vi "send.vi"(8 "error in (no error)":errorcluster, 10 "message":string, 11 "TCPConnection In":refnum<class "TCPConnection.lvclass">) -> (0 "error out":errorcluster, 3 "TCPConnection Out":refnum<class "TCPConnection.lvclass">)   [LabVIEW 2023, in "AbstractFactory.lvlib" / "TCPConnection.lvclass"]
uses:
  TCPConnection.lvclass
  TCPConnection.lvclass/TCPConnection.ctl
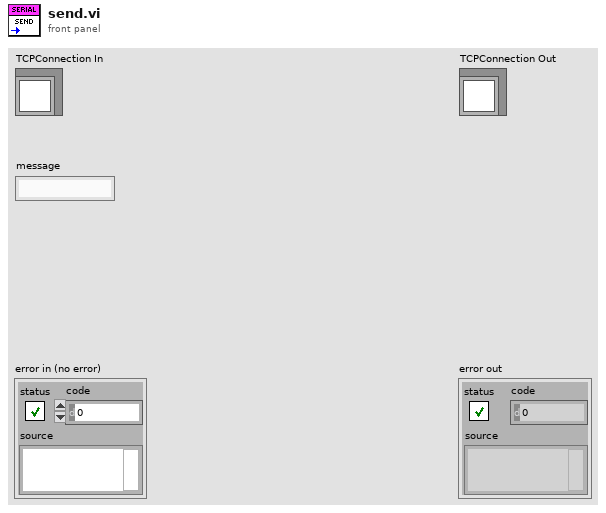
[diagram p1: front panel]
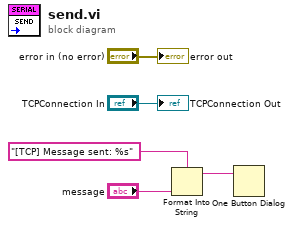
[diagram p0: block diagram]
diagram:
  n1 = Format Into String(format string="[TCP] Message sent: %s", "message") -> (resulting string=w1:string)  [unwired: 2 in, 1 out]
  n2 = One Button Dialog(message=w1) -> ()  [unwired: 1 in, 1 out]
  "error out" <- "error in (no error)"
  "TCPConnection Out" <- "TCPConnection In"
